vi "FPGA_InterruptReadTimestamp.vi"(8 "error in (no error)":errorcluster, 10 "Falling Interrupt":bool, 11 "InteruptRef in":T1) -> (0 "error out":errorcluster, 2 "TimeStamp":u32, 3 "InteruptRef out":T1)   [LabVIEW 2017]
uses:
  <vilib>/Rock Robotics/SystemInterfaces/Interrupt/FPGA_InterruptRef.ctl
  <vilib>/Rock Robotics/SystemInterfaces/Interrupt/FPGA_InterruptIndex.ctl
  <vilib>/rvi/errors/niLvFpgaAdjustHostInterfaceError.vi
  <vilib>/Utility/error.llb/Error Cluster From Error Code.vi
  <vilib>/Rock Robotics/SystemInterfaces/System/FPGA_SystemFPGA Ref Global.vi
  <vilib>/Rock Robotics/SystemInterfaces/System/FPGA_SystemFRC FPGA Ref.ctl
  <vilib>/rvi/interface/nirviReadWriteControl/nirviReadWriteControl.xnode
  NiFpgaLv.dll
  <vilib>/rvi/interface/Simulation/niFpgaSimulationCallBeginRW.vi
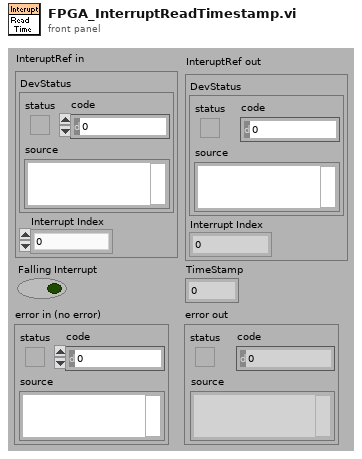
[diagram p1: front panel]
types:
  T1 = typedef "FPGA_InterruptRef.ctl" = cluster{"DevStatus":errorcluster, "Interrupt Index":T2}
  T2 = typedef "FPGA_InterruptIndex.ctl" = enum8{"0", "1", "2", "3", "4", "5", "6", "7", "Invalid"}
  T3 = typedef "FPGA_SystemFRC FPGA Ref.ctl" = refnum<k20>
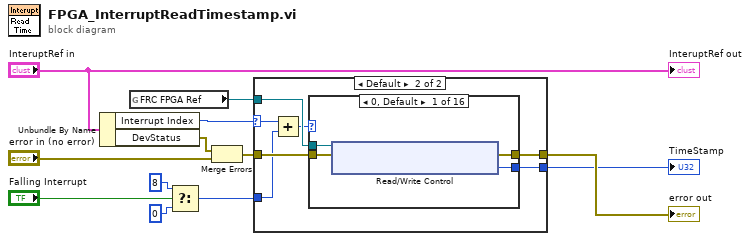
[diagram p0: block diagram]
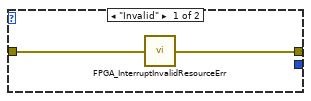
[diagram p2: hidden frame]
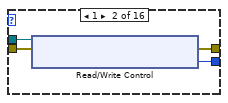
[diagram p3: hidden frame]
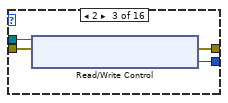
[diagram p4: hidden frame]
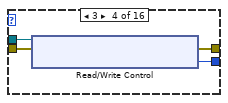
[diagram p5: hidden frame]
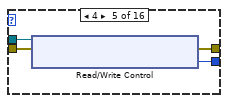
[diagram p6: hidden frame]
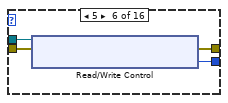
[diagram p7: hidden frame]
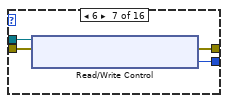
[diagram p8: hidden frame]
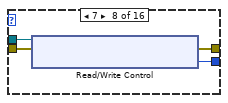
[diagram p9: hidden frame]
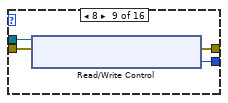
[diagram p10: hidden frame]
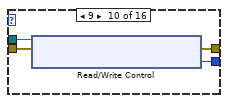
[diagram p11: hidden frame]
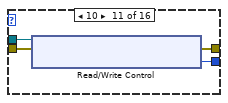
[diagram p12: hidden frame]
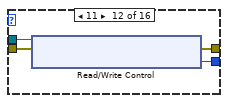
[diagram p13: hidden frame]
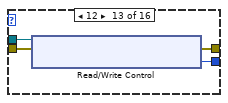
[diagram p14: hidden frame]
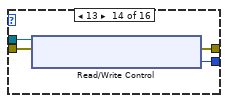
[diagram p15: hidden frame]
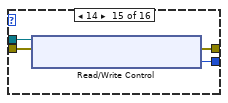
[diagram p16: hidden frame]
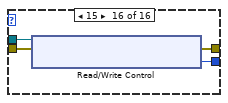
[diagram p17: hidden frame]
diagram:
  n1 = Unbundle By Name("InteruptRef in") -> ("Interrupt Index"=w10:T2, "DevStatus"=w7:errorcluster)
  n2 = global read "FPGA_SystemFPGA Ref Global.vi" "FRC FPGA Ref"() -> (w6:T3)
  n3 = Select(t=8, s="Falling Interrupt", f=0) -> (s? t:f=w4:i32)
  n4 = Merge Errors(w7, "error in (no error)") -> (w9:errorcluster)
  n5 = case shown="Default" w10 {
    selector: w10 -> [_ w19]
    tunnel: [w13 w21] -> w12
    tunnel: [_ w20] -> w11
    tunnel: w9 -> [w14 w18]
    tunnel: w6 -> [_ w17]
    tunnel: w4 -> [_ w15]
    frame "Invalid" {
      n6 = call <vilib>:"FPGA_InterruptInvalidResourceErr.vi"("error in (no error)"=w14) -> ("error out"=w13:errorcluster)
    }
    frame Default {
      n7 = Add(x=w19, y=w15) -> (x+y=w16:i32)
      n8 = case shown="0, Default" w16 {
        tunnel: w17 -> [w24 w29 w33 w37 w41 w45 w49 w53 w57 w61 w65 w69 w73 w77 w81 w85]
        tunnel: w18 -> [w25 w28 w32 w36 w40 w44 w48 w52 w56 w60 w64 w68 w72 w76 w80 w84]
        tunnel: [w23 w27 w31 w35 w39 w43 w47 w51 w55 w59 w63 w67 w71 w75 w79 w83] -> w21
        tunnel: [w22 w26 w30 w34 w38 w42 w46 w50 w54 w58 w62 w66 w70 w74 w78 w82] -> w20
        frame 0, Default {
          n9 = xnode "Read/Write Control"("FPGA VI Reference In"=w24, "error in"=w25) -> ("error out"=w23:errorcluster, "Interrupt0.RisingTimeStamp"=w22:u32)  [unwired: 1 out]
        }
        frame 1 {
          n10 = xnode "Read/Write Control"("FPGA VI Reference In"=w29, "error in"=w28) -> ("error out"=w27:errorcluster, "Interrupt1.RisingTimeStamp"=w26:u32)  [unwired: 1 out]
        }
        frame 2 {
          n11 = xnode "Read/Write Control"("FPGA VI Reference In"=w33, "error in"=w32) -> ("error out"=w31:errorcluster, "Interrupt2.RisingTimeStamp"=w30:u32)  [unwired: 1 out]
        }
        frame 3 {
          n12 = xnode "Read/Write Control"("FPGA VI Reference In"=w37, "error in"=w36) -> ("error out"=w35:errorcluster, "Interrupt3.RisingTimeStamp"=w34:u32)  [unwired: 1 out]
        }
        frame 4 {
          n13 = xnode "Read/Write Control"("FPGA VI Reference In"=w41, "error in"=w40) -> ("error out"=w39:errorcluster, "Interrupt4.RisingTimeStamp"=w38:u32)  [unwired: 1 out]
        }
        frame 5 {
          n14 = xnode "Read/Write Control"("FPGA VI Reference In"=w45, "error in"=w44) -> ("error out"=w43:errorcluster, "Interrupt5.RisingTimeStamp"=w42:u32)  [unwired: 1 out]
        }
        frame 6 {
          n15 = xnode "Read/Write Control"("FPGA VI Reference In"=w49, "error in"=w48) -> ("error out"=w47:errorcluster, "Interrupt6.RisingTimeStamp"=w46:u32)  [unwired: 1 out]
        }
        frame 7 {
          n16 = xnode "Read/Write Control"("FPGA VI Reference In"=w53, "error in"=w52) -> ("error out"=w51:errorcluster, "Interrupt7.RisingTimeStamp"=w50:u32)  [unwired: 1 out]
        }
        frame 8 {
          n17 = xnode "Read/Write Control"("FPGA VI Reference In"=w57, "error in"=w56) -> ("error out"=w55:errorcluster, "Interrupt0.FallingTimeStamp"=w54:u32)  [unwired: 1 out]
        }
        frame 9 {
          n18 = xnode "Read/Write Control"("FPGA VI Reference In"=w61, "error in"=w60) -> ("error out"=w59:errorcluster, "Interrupt1.FallingTimeStamp"=w58:u32)  [unwired: 1 out]
        }
        frame 10 {
          n19 = xnode "Read/Write Control"("FPGA VI Reference In"=w65, "error in"=w64) -> ("error out"=w63:errorcluster, "Interrupt2.FallingTimeStamp"=w62:u32)  [unwired: 1 out]
        }
        frame 11 {
          n20 = xnode "Read/Write Control"("FPGA VI Reference In"=w69, "error in"=w68) -> ("error out"=w67:errorcluster, "Interrupt3.FallingTimeStamp"=w66:u32)  [unwired: 1 out]
        }
        frame 12 {
          n21 = xnode "Read/Write Control"("FPGA VI Reference In"=w73, "error in"=w72) -> ("error out"=w71:errorcluster, "Interrupt4.FallingTimeStamp"=w70:u32)  [unwired: 1 out]
        }
        frame 13 {
          n22 = xnode "Read/Write Control"("FPGA VI Reference In"=w77, "error in"=w76) -> ("error out"=w75:errorcluster, "Interrupt5.FallingTimeStamp"=w74:u32)  [unwired: 1 out]
        }
        frame 14 {
          n23 = xnode "Read/Write Control"("FPGA VI Reference In"=w81, "error in"=w80) -> ("error out"=w79:errorcluster, "Interrupt6.FallingTimeStamp"=w78:u32)  [unwired: 1 out]
        }
        frame 15 {
          n24 = xnode "Read/Write Control"("FPGA VI Reference In"=w85, "error in"=w84) -> ("error out"=w83:errorcluster, "Interrupt7.FallingTimeStamp"=w82:u32)  [unwired: 1 out]
        }
      }
    }
  }
  "error out" <- w12
  "TimeStamp" <- w11
  "InteruptRef out" <- "InteruptRef in"
